vi "generate_x galvo_voltages.vi"(9 "scan specification":T1={"x amplitude"=0, "x resolution (pixels)"=0, "x offset fly-forward (iterations)"=0, "x offset fly-back (iterations)"=0, "y resolution (nr. of lines)"=0, "y step size"=0, "iterations per pixel"=0, "number of frames"=0, "y offset (pixels)"=0, "number of y-brake lines  (before y-fly-back)"=0, "number y-brake lines (after y-fly-back)"=0, "number of y-fly-back steps"=8, "lines per z step"=0, "number of z/intensity tuples"=0, "number of repetitions (volumes or planes)"=0, "z step size derived"=0, "choose the beginning of z scan"=FALSE, "number of frames (settings)"=0, "FPGA trajectory?"=FALSE, "Pockels cell voltage (bits)"=0, "Vy min(bits)"=0, "Vz min(bits)"=0}, 10 "scanning?":bool, 11 "TAG trigger":bool) -> (1 "scanning?":bool, 2 "x galvo voltages":i16)   [LabVIEW 2010]
uses:
  scan_specification_cluster.ctl
panel:
  in  "delay scan start":u16
  in  "iterations until start of fly-back scan segment":u16
  out "counts in last cycle":u16
  out "move galvo?":bool
  out "line ends 2":bool
  in  "TAG trigger 2":bool
  out "control line counter":u16
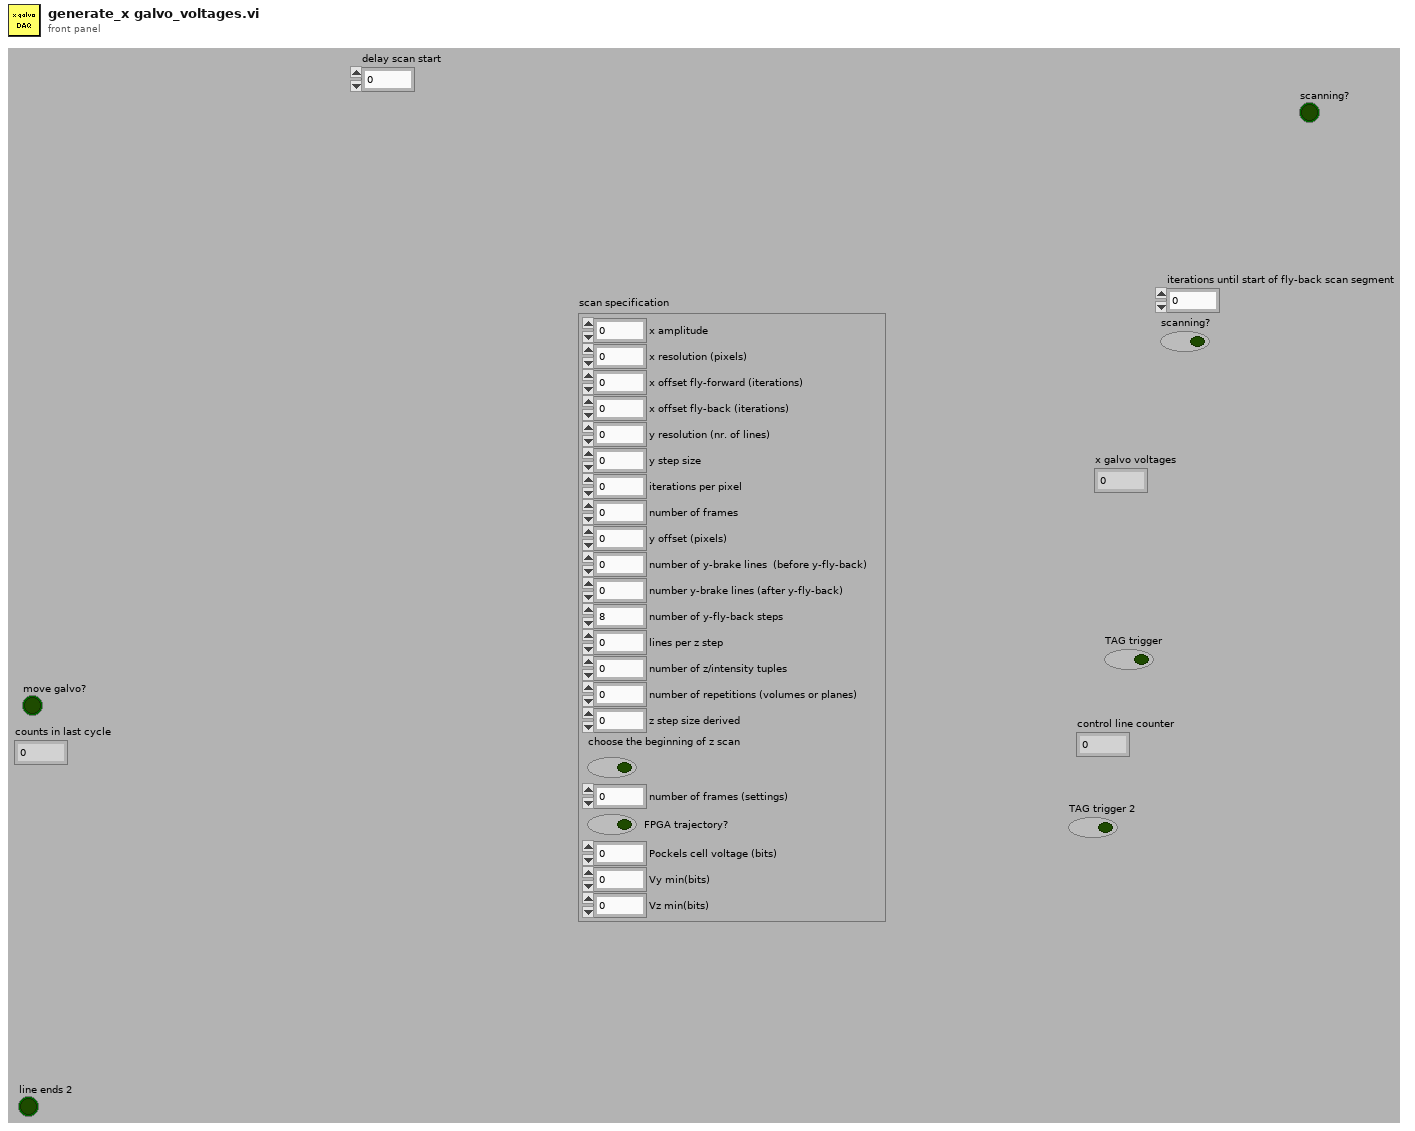
[diagram p1: front panel]
types:
  T1 = typedef "scan_specification_cluster.ctl" = cluster{"x amplitude":u16, "x resolution (pixels)":u16, "x offset fly-forward (iterations)":u16, "x offset fly-back (iterations)":u16, "y resolution (nr. of lines)":u16, "y step size":u16, "iterations per pixel":u16, "number of frames":i32, "y offset (pixels)":u16, "number of y-brake lines  (before y-fly-back)":u16, "number y-brake lines (after y-fly-back)":u16, "number of y-fly-back steps":u16, "lines per z step":u16, "number of z/intensity tuples":u16, "number of repetitions (volumes or planes)":i32, "z step size derived":u16, "choose the beginning of z scan":bool, "number of frames (settings)":i32, "FPGA trajectory?":bool, "Pockels cell voltage (bits)":i16, "Vy min(bits)":i16, "Vz min(bits)":i16}
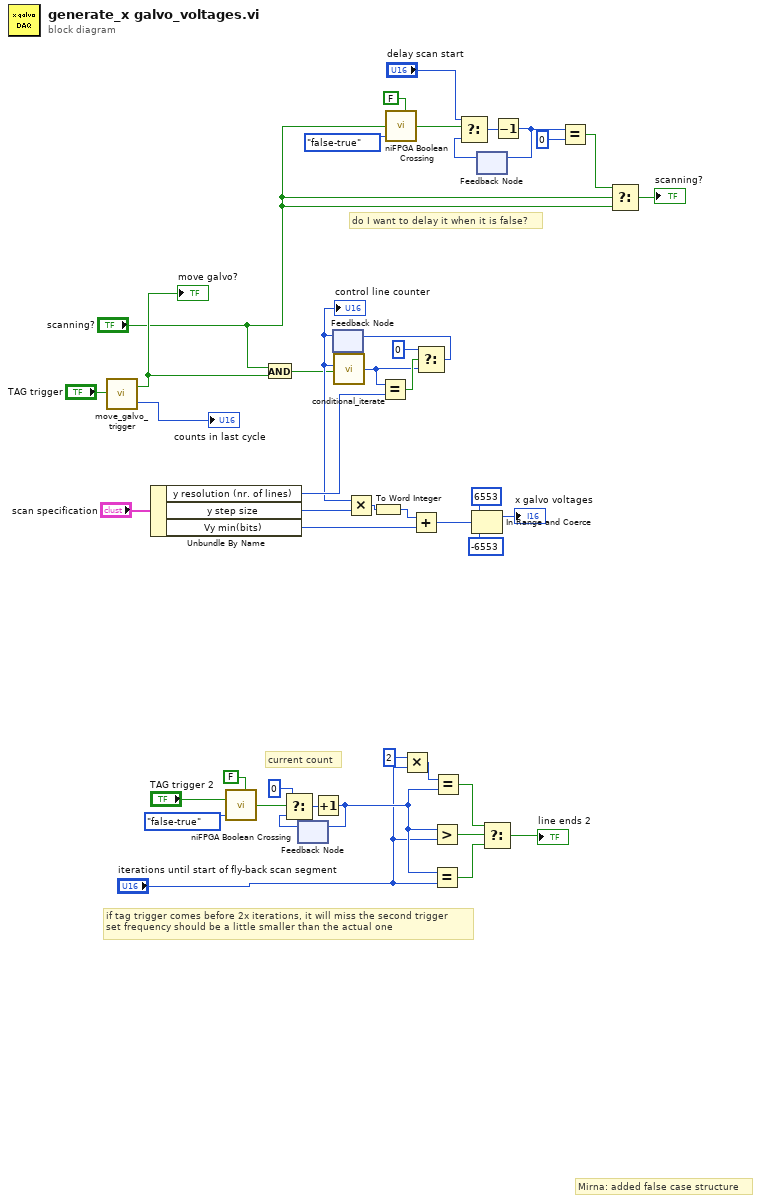
[diagram p0: block diagram]
diagram:
  # "do I want to delay it when it is false?"
  # "if tag trigger comes before 2x iterations, it will miss the second trigger\nset frequency should be a little smaller than the actual one"
  # "current count"
  # "Mirna: added false case structure"
  n1 = call "move_galvo_trigger.vi"("TAG trigger"="TAG trigger") -> ("counts in last cycle"=→"counts in last cycle":u16, ">end of line?>"=w12:bool)
  "move galvo?" <- w12
  n2 = Unbundle By Name("scan specification") -> ("y resolution (nr. of lines)"=w20:u16, "y step size"=w16:u16, "Vy min(bits)"=w18:i16)
  n3 = call <vilib>:"niFPGA Boolean Crossing.vi"("input"="TAG trigger 2", "direction"=enum8{"either", "false-true", "true-false"}."false-true", "initialize"=FALSE) -> ("crossing"=w33:bool)  [unwired: 6 in]
  n4 = And(x="scanning?", y=w12) -> (x .and. y?=w13:bool)
  n5 = feedback #1() -> (w37:u16)  [unwired: 1 in]
  n6 = Select(t=u16 0, s=w33, f=w37) -> (s? t:f=w36:u16)
  n7 = Increment(x=w36) -> (x+1=w28:u16)
  n8 = feedback-in #1(w28) -> ()
  n9 = feedback #2() -> (w17:u16)  [unwired: 1 in]
  "control line counter" <- w17
  n10 = call "conditional_iterate.vi"("iterate?"=w13, "number in"=w17) -> ("number out"=w23:u16)  [unwired: 4 in]
  n11 = Multiply(x=w17, y=w16) -> (x*y=w41:u16)
  n12 = To Word Integer(number=w41) -> (16bit integer=w45:i16)
  n13 = Equal?(x=w23, y=w20) -> (x = y?=w25:bool)
  n14 = call <vilib>:"niFPGA Boolean Crossing.vi"("input"="scanning?", "direction"=enum8{"either", "false-true", "true-false"}."false-true", "initialize"=FALSE) -> ("crossing"=w9:bool)  [unwired: 6 in]
  n15 = Multiply(x=u16 2 ("y"), y="iterations until start of fly-back scan segment") -> (x*y=w29:u16)
  n16 = Add(x=w45, y=w18) -> (x+y=w43:i16)
  n17 = Select(t=u16 0 ("f"), s=w25, f=w23) -> (s? t:f=w22:u16)
  n18 = feedback-in #2(w22) -> ()
  n19 = Greater?(x=w28, y="iterations until start of fly-back scan segment") -> (0:w35:bool)
  n20 = Equal?(x=w28, y="iterations until start of fly-back scan segment") -> (x = y?=w34:bool)
  n21 = Equal?(x=w29, y=w28) -> (x = y?=w27:bool)
  n22 = In Range and Coerce(upper limit=i16 6553, x=w43, lower limit=i16 -6553) -> (coerced(x)=→"x galvo voltages":i16)  [unwired: 1 out]
  n23 = feedback #3() -> (w6:u16)  [unwired: 1 in]
  n24 = Select(t="delay scan start", s=w9, f=w6) -> (s? t:f=w7:u16)
  n25 = Select(t=w27, s=w35, f=w34) -> (s? t:f=→"line ends 2":bool)
  n26 = Decrement(x=w7) -> (x-1=w5:u16)
  n27 = feedback-in #3(w5) -> ()
  n28 = Equal?(x=w5, y=u16 0) -> (x = y?=w1:bool)
  n29 = Select(t=w1, s="scanning?", f="scanning?") -> (s? t:f=→"scanning?":bool)
